vi "DataIsInList.vi"(8 "error in (no error)":errorcluster, 10 "LLNode in":refnum<data-value>, 11 "LinkedList in":refnum<class "LinkedList.lvclass">) -> (0 "error out":errorcluster, 1 "inList":bool, 2 "LLNode out":refnum<data-value>, 3 "LinkedList out":refnum<class "LinkedList.lvclass">, 4 "index":i32)   [LabVIEW 2014, in "LinkedList.lvlib" / "LinkedList.lvclass"]
doc: "Checks to see if the same data of a node is already in the list. This is primarily used to implement graph searches, but could have other uses. You must override LLNode.lvclass:CheckDuplicateData.vi to determine if two nodes have the same data."
uses:
  <userlib>/AdvancedDataStructures/ClassBased/LinkedList/LinkedList.lvclass
  <userlib>/AdvancedDataStructures/ClassBased/LLNode/LLNode.lvclass
  <userlib>/AdvancedDataStructures/ClassBased/LinkedList/LinkedList.lvclass/LinkedList.ctl
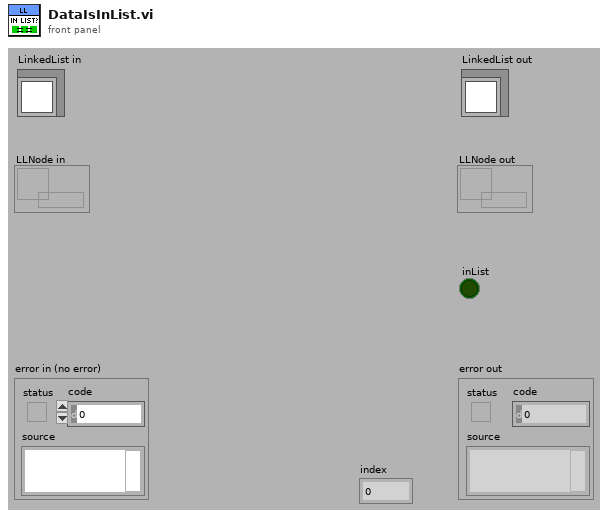
[diagram p1: front panel]
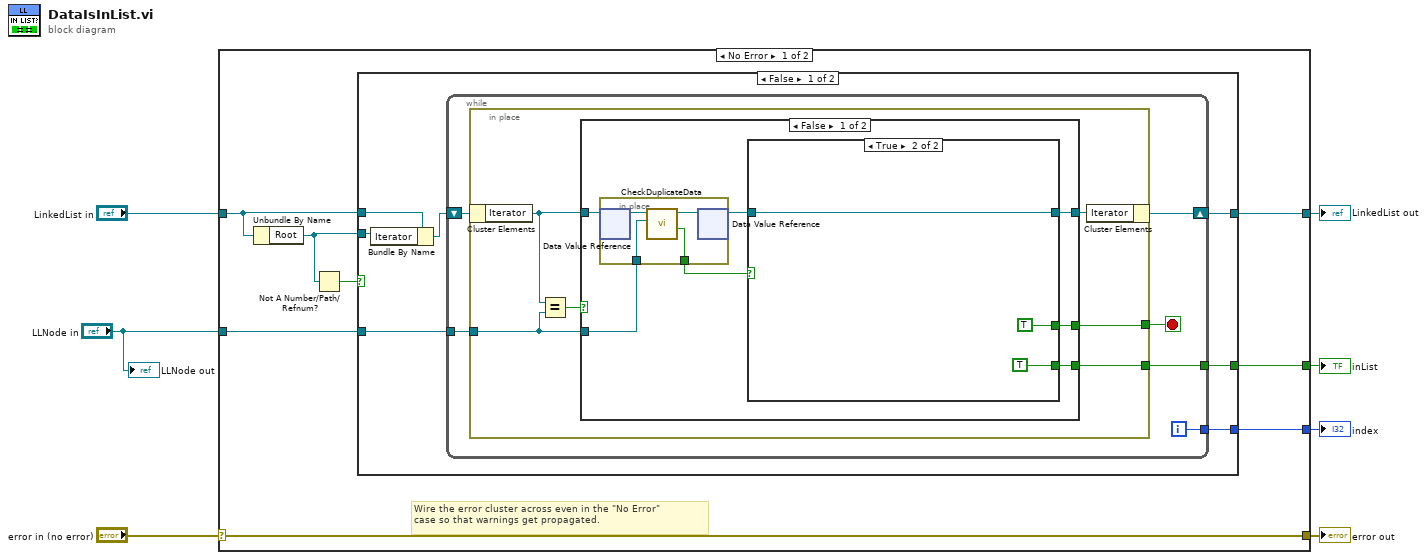
[diagram p0: block diagram]
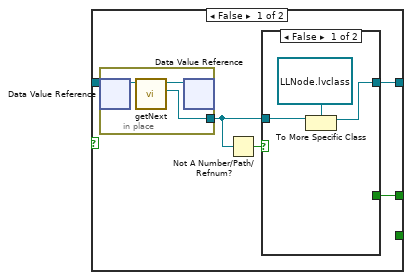
[diagram p2: hidden frame]
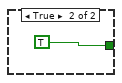
[diagram p3: hidden frame]
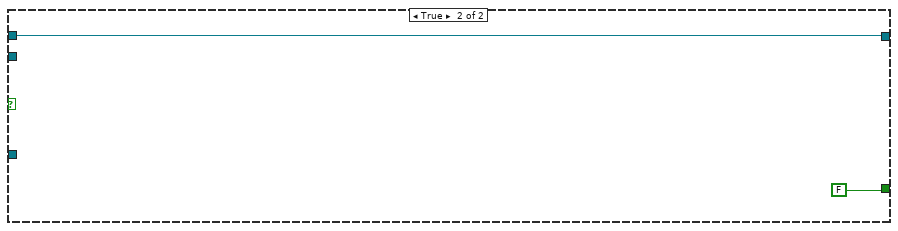
[diagram p5: hidden frame]
diagram:
  n1 = case shown="No Error" "error in (no error)" {
    selector: "error in (no error)" -> [w15 w66]
    tunnel: [w15 w66] -> w6
    tunnel: [w10 w65] -> w4
    tunnel: "LinkedList in" -> [w14 w65]
    tunnel: [w9 _] -> w3
    tunnel: "LLNode in" -> [w11 _]
    tunnel: [w8 _] -> w1
    frame No Error {
      # "Wire the error cluster across even in the \"No Error\"\ncase so that warnings get propagated."
      n2 = Unbundle By Name(w14) -> ("Root"=w13:refnum<data-value>)
      n3 = Not A Number/Path/Refnum?(number/path/refnum=w13) -> (NaN/Path/Refnum?=w12:bool)
      n4 = case shown="False" w12 {
        tunnel: w14 -> [w22 w64]
        tunnel: w13 -> [w21 _]
        tunnel: w11 -> [w19 _]
        tunnel: [w18 w64] -> w10
        tunnel: [w17 FALSE] -> w9
        tunnel: [w16 _] -> w8
        frame False {
          n5 = Bundle By Name(cluster=w22, "Iterator"=w21) -> (w20:refnum<class "LinkedList.lvclass">)
          n6 = while {
            shift-right: [w25] -> w18
            shift-left: w20 -> [w28]
            tunnel: w19 -> [w27]
            tunnel: [w24] -> w17
            tunnel: [w23] -> w16
            i -> [w23]
            stop <- w26 stop-if-true
            n7 = in-place {
              in-place-border: w27 -> [w29]
              in-place-border: [w33] -> w26
              in-place-border: [w31] -> w24
              n8 = in-place-cluster #1(w28) -> ("Iterator"=w30:refnum<data-value>)
              n9 = Equal?(x=w30, y=w29) -> (x = y?=w34:bool)
              n10 = case shown="False" w34 {
                selector: w34 -> [_ w61]
                tunnel: [w41 w61] -> w33
                tunnel: w30 -> [w39 w62]
                tunnel: [w40 w62] -> w32
                tunnel: [w36 w61] -> w31
                tunnel: w29 -> [w35 _]
                frame False {
                  n11 = in-place {
                    in-place-border: [w58] -> w37
                    in-place-border: w35 -> [w57]
                    n12 = in-place-dvr #2(w39) -> (w60:refnum<class "LLNode.lvclass">)  [unwired: 1 out]
                    n13 = call-dynamic "CheckDuplicateData.vi"("ToCheck in"=w57, "LLNode in"=w60) -> ("IsDuplicate"=w58:bool, "LLNode out"=w59:refnum<class "LLNode.lvclass">)  [unwired: 6 in, 2 out]
                    n14 = in-place-dvr #2(w59) -> (w38:refnum<data-value>)  [unwired: 1 out]
                  }
                  n15 = case shown="True" w37 {
                    tunnel: [w44 TRUE] -> w41
                    tunnel: [w43 w54] -> w40
                    tunnel: w38 -> [w42 w54]
                    tunnel: [_ TRUE] -> w36
                    frame False {
                      n16 = in-place {
                        in-place-border: [w51] -> w45
                        n17 = in-place-dvr #3(w42) -> (w53:refnum<class "LLNode.lvclass">)  [unwired: 1 out]
                        n18 = call <userlib>:"getNext.vi"("LLNode in"=w53) -> ("next"=w51:refnum<data-value>, "LLNode out"=w52:refnum<class "LLNode.lvclass">)  [unwired: 8 in, 1 out]
                        n19 = in-place-dvr #3(w52) -> ()  [unwired: 2 out]
                      }
                      n20 = Not A Number/Path/Refnum?(number/path/refnum=w45) -> (NaN/Path/Refnum?=w46:bool)
                      n21 = case shown="False" w46 {
                        tunnel: w45 -> [w49 _]
                        tunnel: [_ TRUE] -> w44
                        tunnel: [w47 _] -> w43
                        frame False {
                          n22 = To More Specific Class(target class=refnum<data-value> refnum ("Iterator"), reference=w49) -> (specific class reference=w47:refnum<data-value>)  [unwired: 1 in, 1 out]
                        }
                        frame True {
                        }
                      }
                    }
                    frame True {
                    }
                  }
                }
                frame True {
                }
              }
              n23 = in-place-cluster #1("Iterator"=w32) -> (w25:refnum<class "LinkedList.lvclass">)
            }
          }
        }
        frame True {
        }
      }
    }
    frame Error {
    }
  }
  "error out" <- w6
  "LinkedList out" <- w4
  "inList" <- w3
  "index" <- w1
  "LLNode out" <- "LLNode in"
